vi "FpgaLink_Write_Channel.vi"(6 "Timeout (10000)":u32, 8 "error in (no error)":errorcluster, 9 "Channel":u8, 10 "data":u8[](array[numeric]), 11 "handle":i64) -> (0 "error out":errorcluster, 3 "handle out":i64)   [LabVIEW 2011]
doc: "Write the supplied data to the specified channel.\n\nrite count bytes from the data array to FPGA channel chan, with the given timeout in milliseconds. In the event of a timeout, the connection between host and FPGA will be left in an undefined state; before the two can resynchronise it's likely the FPGA will need to be reset and the host side disconnected (flOpen()) and reconnected (flClose()) again. Before calling flWriteChannel(), you should verify that the FPGALink device actually supports CommFPGA using flIsCommCapable()."
uses:
  <vilib>/Utility/importsl/GetValueByPointer/datatype.ctl
  <vilib>/Utility/importsl/GetValueByPointer/GetValueByPointer.xnode
  resource/lvimptsl.dll
  libfpgalink.dll
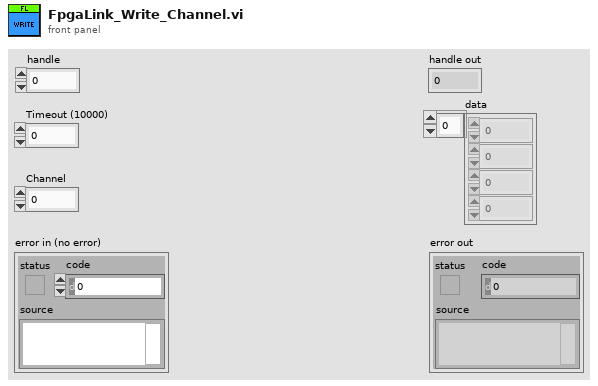
[diagram p1: front panel]
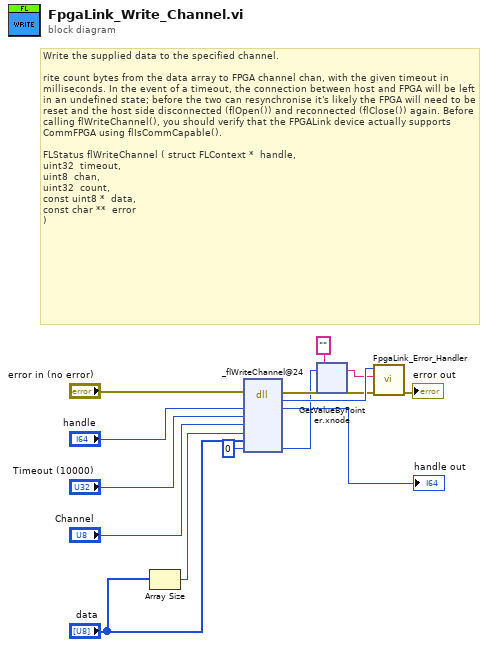
[diagram p0: block diagram]
diagram:
  # "Write the supplied data to the specified channel.\n\nrite count bytes from the data array to FPGA channel chan, with the given timeout in milliseconds. In the event of a timeout, the connection between host and FPGA will be left in an undefined state; before the two can resynchronise it's likely the FPGA will need to be reset and the host side disconnected (flOpen()) and reconnected (flClose()) again. Before calling flWriteChannel(), you should verify that the FPGALink device actually supports CommFPGA using flIsCommCapable().\n\nFLStatus flWriteChannel\t(\tstruct FLContext * \thandle,\nuint32 \ttimeout,\nuint8 \tchan,\nuint32 \tcount,\nconst uint8 * \tdata,\nconst char ** \terror \n)"
  n1 = Array Size(array="data") -> (size(s)=w3:i32)
  n2 = dll-call lib="libfpgalink.*" fn="_flWriteChannel@24"(error in="error in (no error)", "handle"="handle", "timeout"="Timeout (10000)", "chan"="Channel", "count"=w3, "data"="data", "error"=i64 0) -> (error out=w8:errorcluster, "return type"=w11:u32, "handle"=→"handle out":i64, "error"=w7:i64)  [unwired: 6 in, 1 out]
  n3 = xnode "GetValueByPointer.xnode"("Pointer"=w7, "InputType"="", "ErrorIn"=w8) -> ("Output"=w5:string, "ErrorOut"=w9:errorcluster)  [unwired: 1 in]
  n4 = call <vilib>:"FpgaLink_Error_Handler.vi"("error in (no error)"=w9, "error string"=w5, "error code"=w11) -> ("error out"=→"error out":errorcluster)  [unwired: 8 in]
